vi "TEST Blinkin LED selector.vi"() -> ()   [LabVIEW 2023]
uses:
  ctrl defs/ctrl LED PATTERNS.ctl
panel:
  out "pattern\nindex":u16
  out "PWM\npulse\nwidth":dbl
  out "RoboRIO\nSPARK\nvalue":dbl
  in  "Blinkin LED pattern":T1 items=["<<Select a pattern>>", "Rainbow, Rainbow palette", "Rainbow, Party palette", "Rainbow, Ocean palette", "Rainbow, Lava palette", "Rainbow, Forest palette", "Rainbow with glitter", "Confetti", "Shot, Red", "Shot, Blue", "Shot, White", "Sinelon, Rainbow palette", "Sinelon, Party palette", "Sinelon, Ocean palette", "Sinelon, Lava palette", "Sinelon, Forest palette", "BPM, Rainbow palette", "BPM, Party palette", "BPM, Ocean palette", "BPM, Lava palette", "BPM, Forest palette", "Fire, Medium", "Fire, Large", "Twinkles, Rainbow palette", "Twinkles, Party palette", "Twinkles, Ocean palette", "Twinkles, Lava palette", "Twinkles, Forest palette", "Color Waves, Rainbow palette", "Color Waves, Party palette", "Color Waves, Ocean palette", "Color Waves, Lava palette", "Color Waves, Forest palette", "Larson Scanner, Red", "Larson Scanner, Gray", "Light Chase, Red", "Light Chase, Blue", "Light Chase, Gray", "Heartbeat, Red", "Heartbeat, Blue", "Heartbeat, White", "Heartbeat, Gray", "Breath, Red", "Breath, Blue", "Breath, Gray", "Strobe, Red", "Strobe, Blue", "Strobe, Gold", "Strobe, White", "Color 1: End to End Blend to Black", "Color 1: Larson Scanner", "Color 1: Light Chase", "Color 1: Heartbeat Slow", "Color 1: Heartbeat Medium", "Color 1: Heartbeat Fast", "Color 1: Breath Slow", "Color 1: Breath Fast", "Color 1: Shot", "Color 1: Strobe", "Color 2: End to End Blend to Black", "Color 2: Larson Scanner", "Color 2: Light Chase", "Color 2: Heartbeat Slow", "Color 2: Heartbeat Medium", "Color 2: Heartbeat Fast", "Color 2: Breath Slow", "Color 2: Breath Fast", "Color 2: Shot", "Color 2: Strobe", "Color 1/2: Sparkle, 1 on 2", "Color 1/2: Sparkle 2 on 1", "Color 1/2: Gradient", "Color 1/2: BPM", "Color 1/2: End to End Blend 1 to 2", "Color 1/2: End to End Blend 2 to 1", "Color 1/2: setup pattern", "Color 1/2: Twinkles", "Color 1/2: Color Waves", "Color 1/2: Sinelon", "Solid Hot Pink", "Solid Dark Red", "Solid Red", "Solid Red Orange", "Solid Orange", "Solid Gold", "Solid Yellow", "Solid Lawn Green", "Solid Lime", "Solid Dark Green", "Solid Green", "Solid Blue Green", "Solid Aqua", "Solid Sky Blue", "Solid Dark Blue", "Solid Blue", "Solid Blue Violet", "Solid Violet", "Solid White", "Solid Gray", "Solid Dark Gray", "Solid Black"]
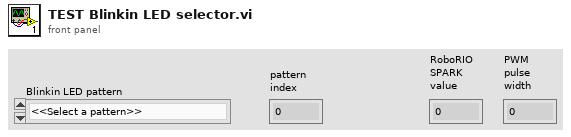
[diagram p1: front panel]
types:
  T1 = typedef "ctrl LED PATTERNS.ctl" = u16
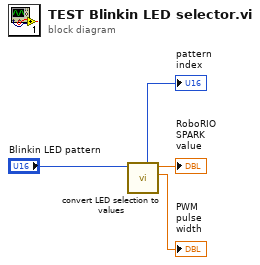
[diagram p0: block diagram]
diagram:
  n1 = call "convert LED selection to values.vi"("Blinkin LED pattern"="Blinkin LED pattern") -> ("PULSE value"=→"PWM\npulse\nwidth":dbl, "SPARK value"=→"RoboRIO\nSPARK\nvalue":dbl, "pattern\nindex"=→"pattern\nindex":u16)  [unwired: 8 in]
